vi "Read.vi"(8 "error in (no error)":errorcluster, 11 "Numeric Array in":refnum<class "Double Float Array 1D.lvclass">) -> (0 "error out":errorcluster, 2 "Numeric":dbl, 3 "Numeric Array out":refnum<class "Double Float Array 1D.lvclass">)   [LabVIEW 2021, in "Variable.lvlib" / "Double Float Array 1D.lvclass"]
uses:
  Double Float Array 1D.lvclass
  C:/Users/Tim/Documents/LabVIEW/2021/Data Classes/Source/Element/Vector Parent/Vector Parent.lvclass
  Element/Vector Parent/Vector Parent.lvclass/Vector Parent.ctl
  Double Float Array 1D.lvclass/Double Float Array 1D.ctl
  Element/Vector Parent/Properties/Read Index.vi
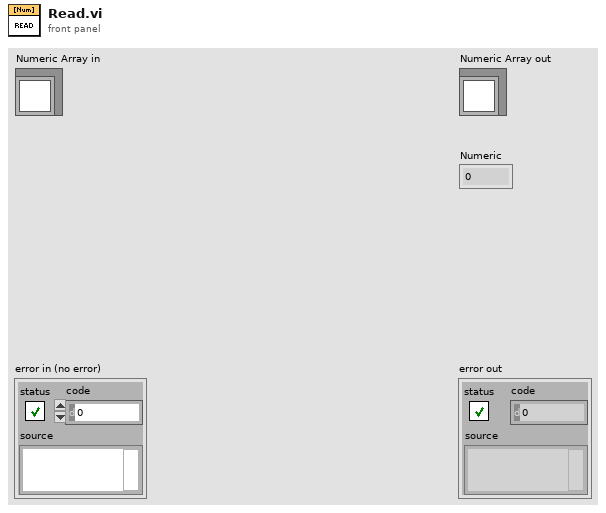
[diagram p1: front panel]
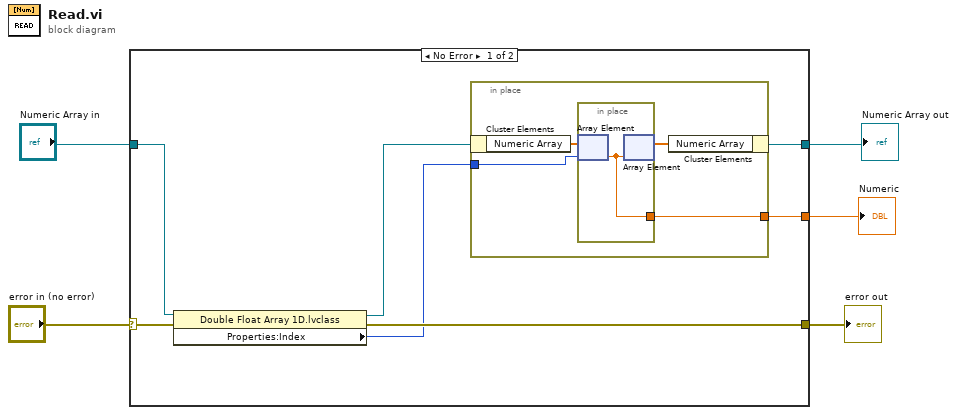
[diagram p0: block diagram]
diagram:
  n1 = case shown="No Error" "error in (no error)" {
    selector: "error in (no error)" -> [w10 w19]
    tunnel: [w7 w19] -> w2
    tunnel: "Numeric Array in" -> [w9 w18]
    tunnel: [w12 w18] -> w4
    tunnel: [w11 _] -> w3
    frame No Error {
      n2 = property class="Double Float Array 1D.lvclass"(reference=w9, error in=w10) -> (reference out=w8:refnum<class "Double Float Array 1D.lvclass">, error out=w7:errorcluster, "Properties:Index"=w6:i32)
      n3 = in-place {
        in-place-border: w6 -> [w15]
        in-place-border: [w13] -> w11
        n4 = in-place-cluster #1(w8) -> ("Numeric Array"=w16:dbl[])
        n5 = in-place {
          in-place-border: [w17] -> w13
          n6 = in-place-array #2(w16, w15) -> (w17:dbl)
          n7 = in-place-array #2(w17) -> (w14:dbl[])  [unwired: 1 out]
        }
        n8 = in-place-cluster #1("Numeric Array"=w14) -> (w12:refnum<class "Double Float Array 1D.lvclass">)
      }
    }
    frame Error {
    }
  }
  "error out" <- w2
  "Numeric Array out" <- w4
  "Numeric" <- w3
